vi "LaunchClient.vi"   [LabVIEW 2023]
uses:
  TCP_Client/TCP_Client.lvclass
  <vilib>/ActorFramework/Actor/Actor.lvclass
  C:/Program Files (x86)/National Instruments/LabVIEW 2023/vi.lib/ActorFramework/Actor/Actor.lvclass
  C:/Source/LabVIEW/TCP_server/TCP_Client/TCP_Client/TCP_Client.lvclass
  C:/Source/LabVIEW/TCP_server/SimpleErrorLogger/ApplicationWithErrorLogger/ApplicationWithErrorLogger.lvclass
types:
  T1 = enum32{"Invalid", "Standard", "Closed", "Hidden", "Minimized", "Maximized"}
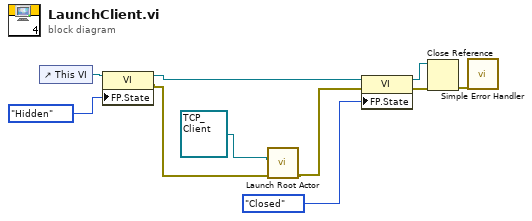
[diagram p0: block diagram]
diagram:
  n1 = control-ref of="This VI"() -> (w9:refnum<vi>)
  n2 = property class="VI"(reference=w9, "FP.State"=T1."Hidden" ("Front Panel Window:State")) -> (reference out=w5:refnum<vi>, error out=w7:errorcluster)  [unwired: 1 in]
  n3 = call <vilib>:"Launch Root Actor.vi"("error in (no error)"=w7, "Actor"=refnum<class "TCP_Client.lvclass"> refnum ("TCP_Client.lvlib:TCP_Client.lvclass")) -> ("error out"=w6:errorcluster)  [unwired: 8 in, 1 out]
  n4 = property class="VI"(reference=w5, error in=w6, "FP.State"=T1."Closed" ("Front Panel Window:State")) -> (reference out=w2:refnum<vi>, error out=w3:errorcluster)
  n5 = Close Reference(reference=w2, error in (no error)=w3) -> (error out=w1:errorcluster)
  n6 = call <vilib>:"Simple Error Handler.vi"("error in (no error)"=w1) -> ()  [unwired: 4 in, 5 out]
